vi "GSP_Manager_COLL.vi"() -> ()   [LabVIEW 2015]
uses:
  SystemUtil/ScriptArray.ctl
  SystemUtil/Script.ctl
  SystemUtil/Command.ctl
  SystemUtil/MotorStates.ctl
  SystemUtil/ThreadStates.ctl
  Log/LogItem.ctl
  GSP_COLL_Global.vi
  GUI/GSP_GUI_global.vi
panel:
  in  "Change Coll":bool
  out "Coll Actual":i32 caption="Actual"
  in  "Coll Target":i32 caption="Target" min=-4000 max=1000
  out "Coll Ext Temp":dbl(slide) scale=0.0..20.0
  out "Last Error":errorcluster
  in  "CommandQ":string
  # "Collimator Focus"
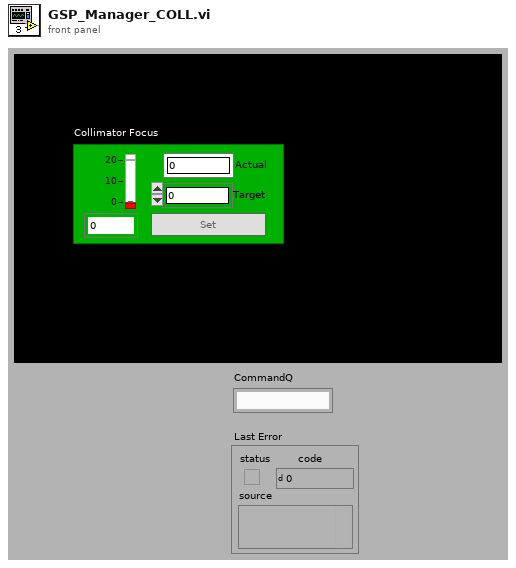
[diagram p1: front panel]
types:
  T1 = typedef "Command.ctl" = cluster{"Command":string, "Parameter":string}
  T2 = typedef "ScriptArray.ctl" = T3[]
  T3 = typedef "Script.ctl" = cluster{"Current Step":i32, "Commands":cluster{"Command":string, "Parameters":string}[]}
  T4 = cluster{"Move Mem Address":i32, "Home Mem Address":i32}
  T5 = enum16{"POL (0)", "CPL (1)", "HLT (2)", "STP (3)", "RST (4)", "RVN (5)", "RPB (6)", "CLP (8)", "SDL (9)", "RUN (10)", "WRI (11)", "RRG (12)", "SPR (13)", "LPR (14)", "VMI (15)", "SSP (17)", "SSE (18)", "RIS (20)", "RIO (21)", "IMW (25)", "END (128)", "MAV (134)", "MRV (135)", "JRE (137)", "WCL (138)", "WCW (139)", "DLY (140)", "WDL (141)", "GCL (142)", "GOP (143)", "ZTG (144)", "ZTP (145)", "TTP (146)", "CME (147)", "CTC (148)", "TQL (149)", "AHC (150)", "ERL (151)", "OLP (152)", "WRP (154)", "IDT (155)", "LRP (156)", "VMP (159)", "RAV (160)", "RRV (161)", "JMP (162)", "JOI (162)", "CIS (163)", "CKS (164)", "CLC (165)", "KMC (167)", "MCT (168)", "FLC (169)", "EEM (170)", "DDB (171)", "DEM (171)", "PAC (172)", "ADL (173)", "BRT (174)", "MAT (176)", "MRT (177)", "RAT (178)", "RRT (179)", "SSD (180)", "KMR (181)", "KED (182)", "KDD (183)", "DIR (184)", "PRO (185)", "SIF (186)", "EDL (187)", "CIO (188)", "MDS (189)", "MDC (190)", "MDT (191)", "SEE (192)", "ARI (193)", "WBS (194)", "SCF (195)", "RSM (196)", "RLM (197)", "RSN (198)", "RLN (199)", "PCL (201)", "PCI (201)", "PRT (202)", "PRI (202)", "WBE (204)", "SOB (205)", "COB (206)", "ACR (207)", "PLR (208)", "CAI (211)", "LVT (212)", "OVT (213)", "MTT (214)", "CLC (215)", "PIM (216)", "VIM (217)", "TIM (218)", "AHM (219)", "SSL (221)", "TRU (222)", "RSD (223)", "EMT (225)", "DMT (226)", "EMD (227)", "DMD (228)", "HSM (229)", "AHD (230)", "PCM (231)", "PCG (232)", "XRV (233)", "XAV (234)", "XRT (235)", "XAT (236)", "GOC (237)", "JNA (238)", "JOR (239)", "PMC (240)", "PMV (241)", "PMX (242)", "DLC (243)", "SLC (244)", "PCP (245)", "ATR (248)", "PMO (249)", "JAN (250)", "EDH (251)", "DIF (252)", "IMS (253)", "IMQ (254)"}
  T6 = typedef "MotorStates.ctl" = enum16{"Ready", "Moving", "Uninitialized", "Error"}
  T7 = typedef "ThreadStates.ctl" = enum16{"Waiting", "Scripting", "Uninitialized", "Error"}
  T8 = enum16{"Launch", "Log", "Open", "Close", "Shutdown"}
  T9 = typedef "LogItem.ctl" = cluster{"error in (no error)":errorcluster, "Source":string, "Comment ":string}
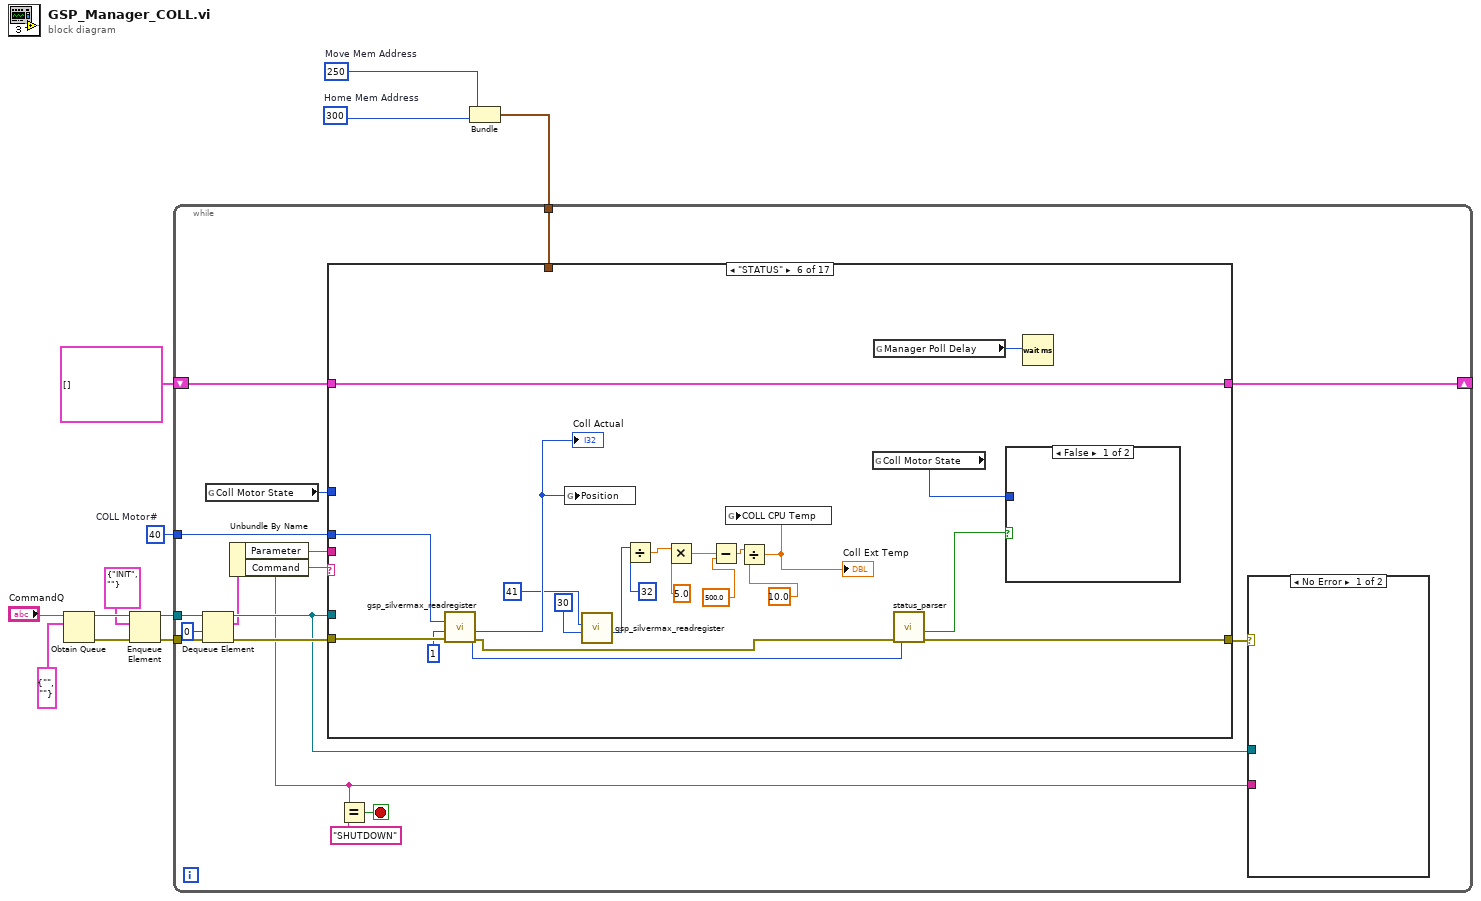
[diagram p0: block diagram]
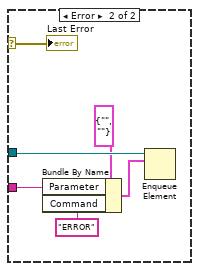
[diagram p2: hidden frame]
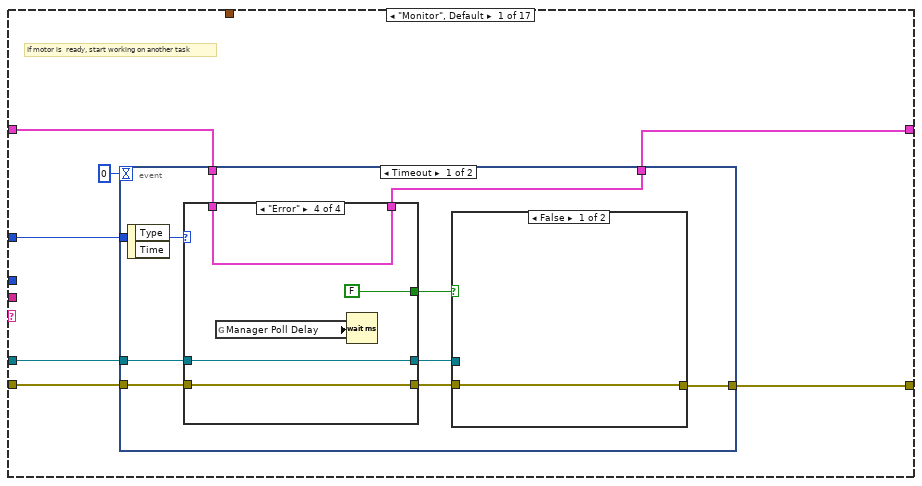
[diagram p3: hidden frame]
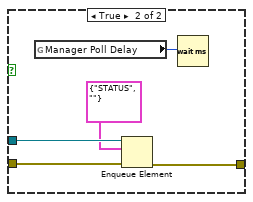
[diagram p4: hidden frame]
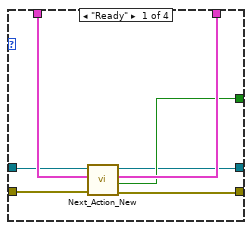
[diagram p5: hidden frame]
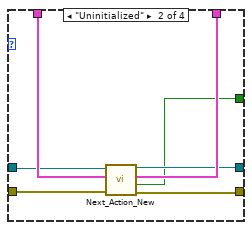
[diagram p6: hidden frame]
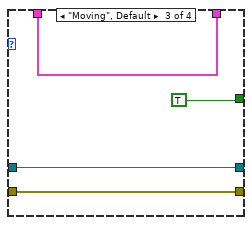
[diagram p7: hidden frame]
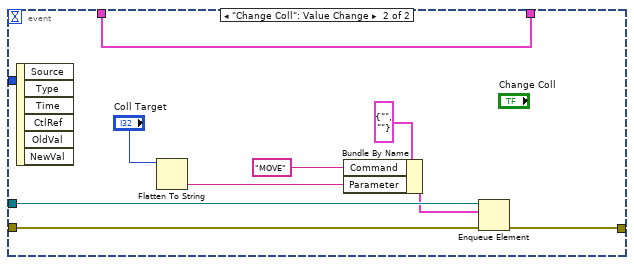
[diagram p8: hidden frame]
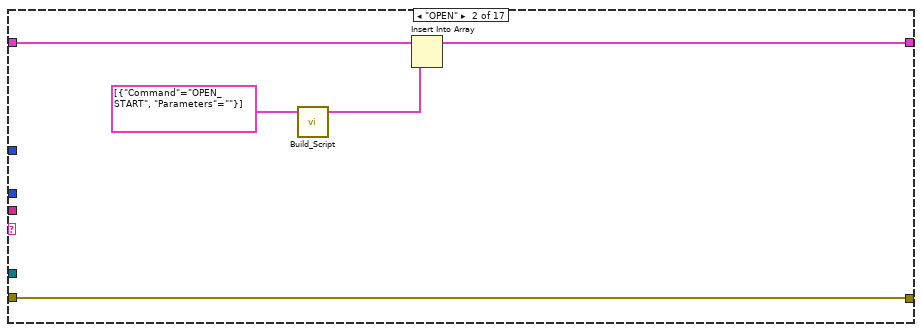
[diagram p9: hidden frame]
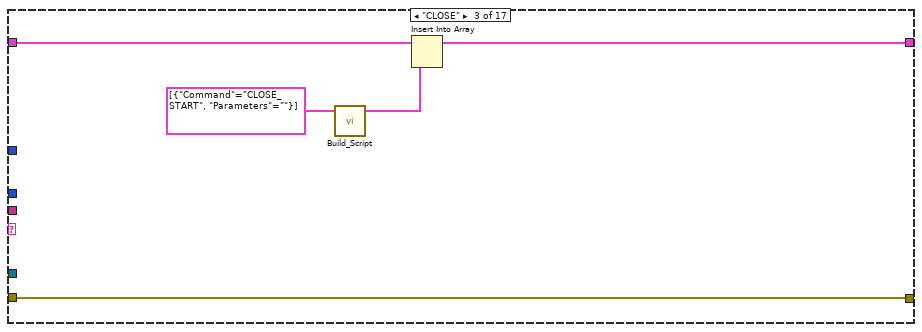
[diagram p10: hidden frame]
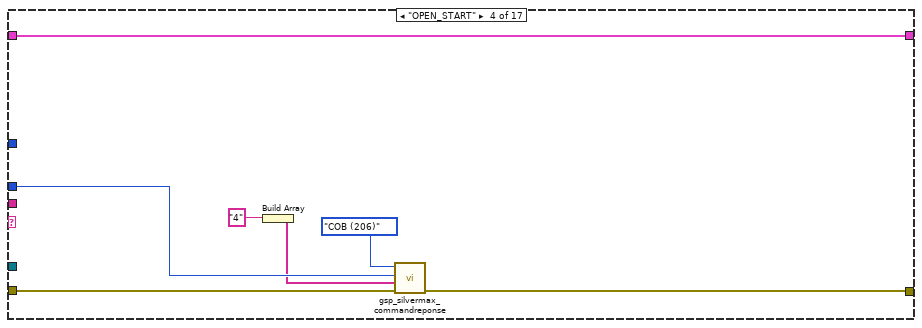
[diagram p11: hidden frame]
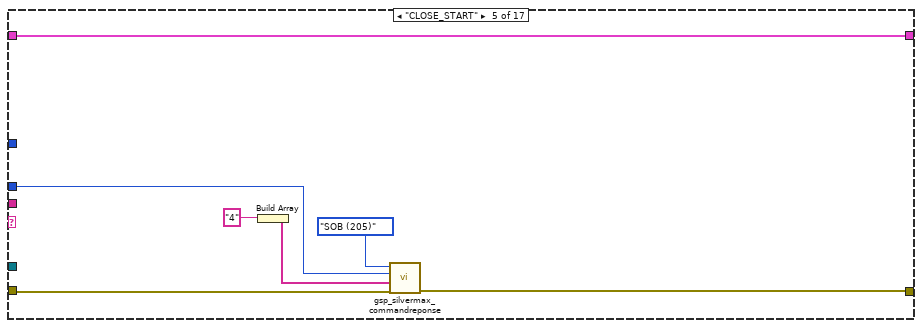
[diagram p12: hidden frame]
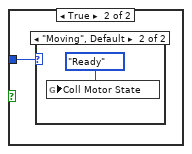
[diagram p13: hidden frame]
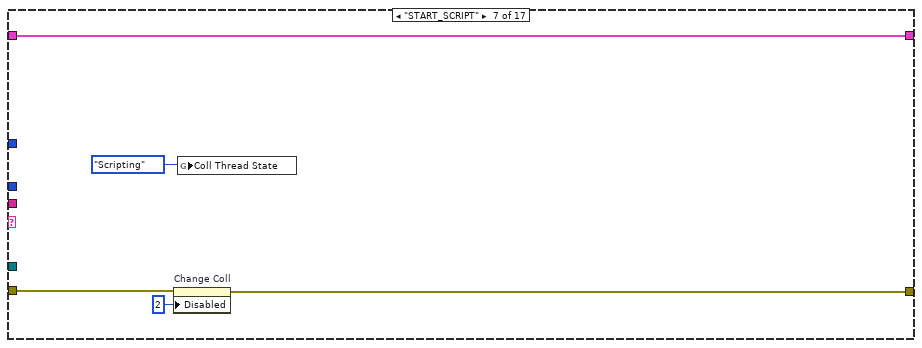
[diagram p15: hidden frame]
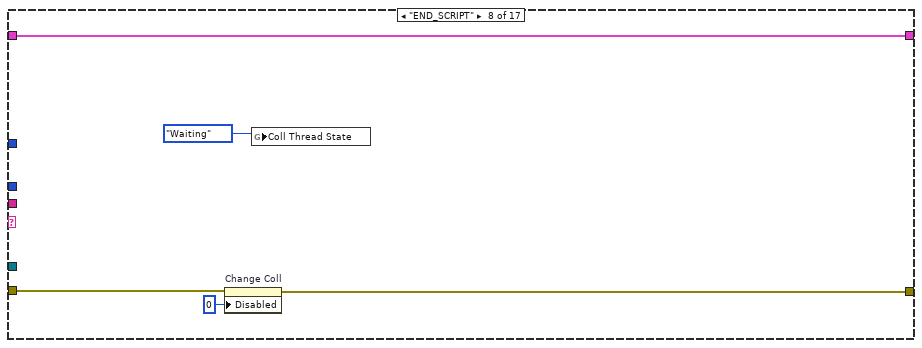
[diagram p16: hidden frame]
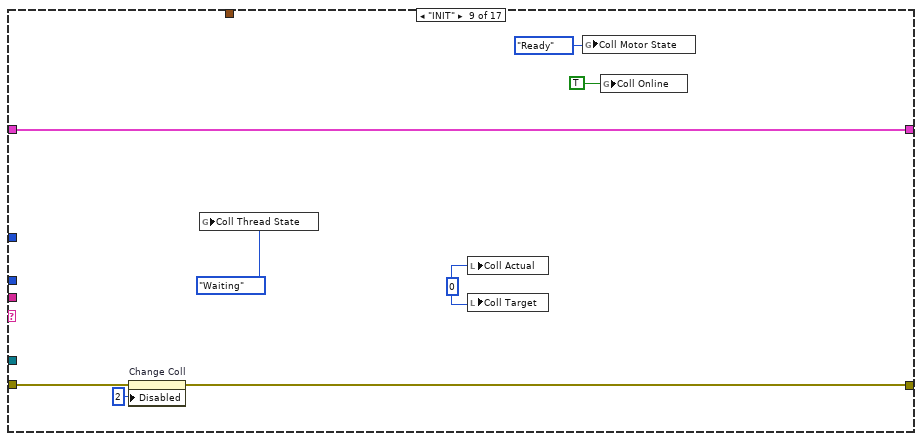
[diagram p17: hidden frame]
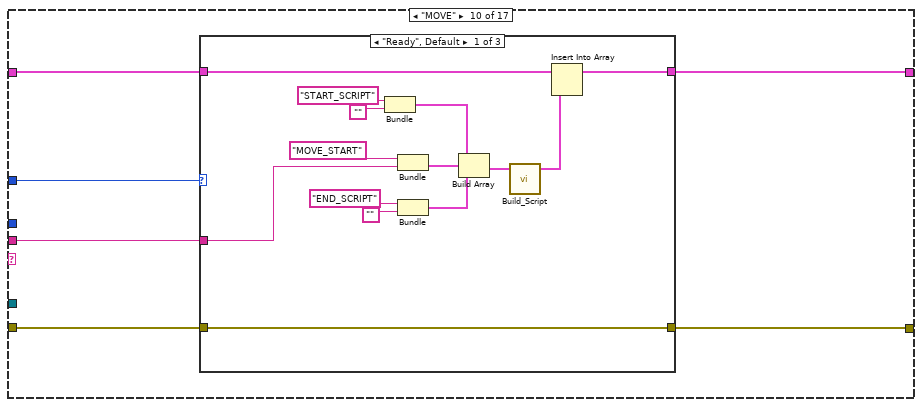
[diagram p18: hidden frame]
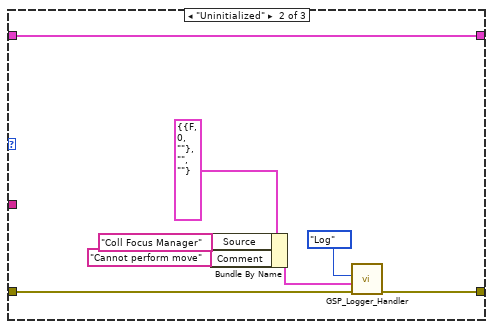
[diagram p19: hidden frame]
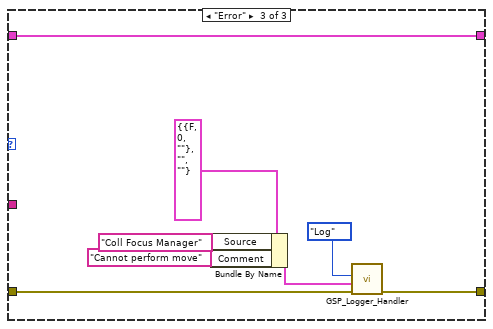
[diagram p20: hidden frame]
diagram:
  w2 = 300  # Home Mem Address
  w3 = 250  # Move Mem Address
  w4 = u8 40  # COLL Motor#
  n1 = Obtain Queue(name (unnamed)="CommandQ", element data type=T1 {"Command"="", "Parameter"=""} ("Command")) -> (queue out=w9:refnum<queue>, error out=w10:errorcluster)  [unwired: 3 in, 1 out]
  n2 = Enqueue Element(queue=w9, element=T1 {"Command"="INIT", "Parameter"=""}, error in (no error)=w10) -> (queue out=w12:refnum<queue>, error out=w11:errorcluster)  [unwired: 1 in, 1 out]
  n3 = Bundle("Move Mem Address"=w3, "Home Mem Address"=w2) -> (w1:T4)  [unwired: 1 in]
  n4 = while {
    tunnel: w12 -> [w28]
    tunnel: w11 -> [w27]
    tunnel: w4 -> [w22]
    shift-right: [w21] -> _
    shift-left: T2 [] ("Operations") -> [w20]
    tunnel: w1 -> [w13]
    stop <- w16 stop-if-true
    n5 = Dequeue Element(queue=w28, timeout in ms (-1)=0, error in (no error)=w27) -> (queue out=w24:refnum<queue>, element=w18:T1, error out=w26:errorcluster)  [unwired: 1 out]
    n6 = global read "GSP_COLL_Global.vi" "Coll Motor State"() -> (w14:T6)
    n7 = Unbundle By Name(w18) -> ("Parameter"=w17:string, "Command"=w15:string)
    n8 = case shown="\"STATUS\"" w15 {
      tunnel: w26 -> [w40 w91 w96 w104 w108 w134 w140 w145 w151 w157 w191 w214 w220 w223 w238 w242 _]
      tunnel: w24 -> [w41 _ _ _ _ _ _ _ _ _ _ w215 _ _ _ _ w251]
      tunnel: [w36 w91 w96 w102 w107 w131 w138 w143 w147 w156 w201 w212 w220 w229 w237 w241 _] -> w25
      tunnel: w22 -> [_ _ _ w100 w106 w133 _ _ _ _ w195 _ _ w232 _ _ _]
      tunnel: w20 -> [w39 w93 w98 w105 w112 w129 w141 w146 w153 w160 w198 w216 w222 w226 w239 w243 w246]
      tunnel: [w38 w92 w97 w105 w112 w129 w141 w146 w153 w159 w198 w216 w221 w226 w239 w243 w245] -> w21
      tunnel: w17 -> [_ _ _ _ _ _ _ _ _ w158 w196 _ _ _ _ _ _]
      tunnel: w14 -> [w37 _ _ _ _ _ _ _ _ w155 _ _ _ _ _ _ _]
      tunnel: w13 -> [_ _ _ _ _ _ _ _ _ _ w194 _ _ w225 _ _ _]
      frame "Monitor", Default {
        # "If motor is  ready, start working on another task"
        n9 = event shown="[0] Timeout" {
          selector: _ -> [_ _]
          dyn-events: _ -> [_ _]
          timeout: 0 -> [_ _]
          tunnel: w41 -> [w50 w83]
          tunnel: w40 -> [w49 w82]
          tunnel: w39 -> [w48 w88]
          tunnel: [w47 w88] -> w38
          tunnel: w37 -> [w46 _]
          tunnel: [w43 w81] -> w36
          event Timeout {
            n10 = event-data() -> ()  [unwired: 1 in, 2 out]
            n11 = case shown="\"Error\"" w46 {
              tunnel: w50 -> [w59 w66 w72 w76]
              tunnel: w49 -> [w63 w70 w73 w78]
              tunnel: [w61 w68 w73 w78] -> w45
              tunnel: w48 -> [w62 w69 w74 w79]
              tunnel: [w60 w67 w74 w79] -> w47
              tunnel: [w57 w65 w72 w76] -> w44
              tunnel: [w58 w64 TRUE FALSE] -> w42
              frame "Ready" {
                n12 = call "Next_Action_New.vi"("error in (no error)"=w63, "Operations"=w62, "queue in"=w59) -> ("error out"=w61:errorcluster, "No command?"=w58:bool, "Operations Out"=w60:T2, "queue out"=w57:refnum<queue>)  [unwired: 1 in]
              }
              frame "Uninitialized" {
                n13 = call "Next_Action_New.vi"("error in (no error)"=w70, "Operations"=w69, "queue in"=w66) -> ("error out"=w68:errorcluster, "No command?"=w64:bool, "Operations Out"=w67:T2, "queue out"=w65:refnum<queue>)  [unwired: 1 in]
              }
              frame "Moving", Default {
              }
              frame "Error" {
                n14 = global read "GSP_GUI_global.vi" "Manager Poll Delay"() -> (w77:u32)
                n15 = Wait (ms)(milliseconds to wait=w77) -> ()  [unwired: 1 out]
              }
            }
            n16 = case shown="False" w42 {
              tunnel: w45 -> [w51 w56]
              tunnel: w44 -> [_ w55]
              tunnel: [w51 w54] -> w43
              frame False {
              }
              frame True {
                n17 = global read "GSP_GUI_global.vi" "Manager Poll Delay"() -> (w53:u32)
                n18 = Enqueue Element(queue=w55, element=T1 {"Command"="STATUS", "Parameter"=""}, error in (no error)=w56) -> (error out=w54:errorcluster)  [unwired: 1 in, 2 out]
                n19 = Wait (ms)(milliseconds to wait=w53) -> ()  [unwired: 1 out]
              }
            }
          }
          event "Change Coll": Value Change {
            n20 = event-data() -> ()  [unwired: 1 in, 6 out]
            n21 = Flatten To String(anything="Coll Target") -> (data string=w85:string)  [unwired: 3 in, 2 out]
            n22 = Bundle By Name(cluster=T1 {"Command"="", "Parameter"=""} ("element"), "Command"="MOVE" ("element"), "Parameter"=w85) -> (w80:T1)
            n23 = Enqueue Element(queue=w83, element=w80, error in (no error)=w82) -> (error out=w81:errorcluster)  [unwired: 1 in, 2 out]
          }
        }
      }
      frame "OPEN" {
        n24 = call "Build_Script.vi"("Commands"=cluster{"Command":string, "Parameters":string}[] [{"Command"="OPEN_START", "Parameters"=""}]) -> ("script out"=w90:T3)  [unwired: 4 in]
        n25 = Insert Into Array(array=w93, new element=w90) -> (w92:T2)  [unwired: 1 in]
      }
      frame "CLOSE" {
        n26 = call "Build_Script.vi"("Commands"=cluster{"Command":string, "Parameters":string}[] [{"Command"="CLOSE_START", "Parameters"=""}]) -> ("script out"=w95:T3)  [unwired: 4 in]
        n27 = Insert Into Array(array=w98, new element=w95) -> (w97:T2)  [unwired: 1 in]
      }
      frame "OPEN_START" {
        n28 = Build Array("4") -> (w99:string[])
        n29 = call "gsp_silvermax_commandreponse.vi"("error in (no error)"=w104, "Parameters (none)"=w99, "Motor #"=w100, "Command"=T5."COB (206)") -> ("error out"=w102:errorcluster)  [unwired: 3 out]
      }
      frame "CLOSE_START" {
        n30 = Build Array("4") -> (w109:string[])
        n31 = call "gsp_silvermax_commandreponse.vi"("error in (no error)"=w108, "Parameters (none)"=w109, "Motor #"=w106, "Command"=T5."SOB (205)") -> ("error out"=w107:errorcluster)  [unwired: 3 out]
      }
      frame "STATUS" {
        n32 = call "gsp_silvermax_readregister.vi"("error in (no error)"=w134, "Register# (0)"=u8 1, "Motor #"=w133) -> ("error out"=w113:errorcluster, "Register Value"=w121:i32, "Motor # dup"=w114:u8)  [unwired: 2 in, 2 out]
        "Coll Actual" <- w121
        n33 = global write "GSP_COLL_Global.vi" "Position"(w121) -> ()
        n34 = call "gsp_silvermax_readregister.vi"("Register# (0)"=u8 30, "Motor #"=41) -> ("Register Value"=w123:i32)  [unwired: 3 in, 4 out]
        n35 = Divide(x=w123, y=32) -> (x/y=w125:dbl)
        n36 = Multiply(x=w125, y=5.0) -> (x*y=w120:dbl)
        n37 = Subtract(x=w120, y=500.0) -> (x-y=w119:dbl)
        n38 = Divide(x=w119, y=10.0) -> (x/y=w117:dbl)
        "Coll Ext Temp" <- w117
        n39 = global write "GSP_COLL_Global.vi" "COLL CPU Temp"(w117) -> ()
        n40 = global read "GSP_COLL_Global.vi" "Coll Motor State"() -> (w122:T6)
        n41 = global read "GSP_GUI_global.vi" "Manager Poll Delay"() -> (w128:u32)
        n42 = call "status_parser.vi"("error in (no error)"=w113, "Motor #"=w114) -> ("error out"=w131:errorcluster, "Program Complete?"=w130:bool)  [unwired: 3 in, 1 out]
        n43 = case shown="False" w130 {
          tunnel: w122 -> [_ w135]
          frame False {
          }
          frame True {
            n44 = case shown="\"Moving\", Default" w135 {
              frame "Uninitialized" {
              }
              frame "Moving", Default {
                n45 = global write "GSP_COLL_Global.vi" "Coll Motor State"(MotorStates."Ready" ("Mode")) -> ()
              }
            }
          }
        }
        n46 = Wait (ms)(milliseconds to wait=w128) -> ()  [unwired: 1 out]
      }
      frame "START_SCRIPT" {
        n47 = property on="Change Coll" class="Bool"(error in=w140, "Disabled"=u8 2) -> (error out=w138:errorcluster)  [unwired: 1 in, 1 out]
        n48 = global write "GSP_COLL_Global.vi" "Coll Thread State"(ThreadStates."Scripting" ("Thread state")) -> ()
      }
      frame "END_SCRIPT" {
        n49 = property on="Change Coll" class="Bool"(error in=w145, "Disabled"=u8 0) -> (error out=w143:errorcluster)  [unwired: 1 in, 1 out]
        n50 = global write "GSP_COLL_Global.vi" "Coll Thread State"(ThreadStates."Waiting" ("Thread state")) -> ()
      }
      frame "INIT" {
        w150 = 0 ("Value")
        n51 = property on="Change Coll" class="Bool"(error in=w151, "Disabled"=u8 2) -> (error out=w147:errorcluster)  [unwired: 1 in, 1 out]
        n52 = global write "GSP_COLL_Global.vi" "Coll Thread State"(ThreadStates."Waiting" ("Thread state")) -> ()
        n53 = local write "Coll Actual"(w150) -> ()
        n54 = local write "Coll Target"(w150) -> ()
        n55 = global write "GSP_COLL_Global.vi" "Coll Motor State"(MotorStates."Ready" ("Mode")) -> ()
        n56 = global write "GSP_COLL_Global.vi" "Coll Online"(TRUE ("CS Online")) -> ()
      }
      frame "MOVE" {
        n57 = case shown="\"Ready\", Default" w155 {
          tunnel: w160 -> [w174 w176 w184]
          tunnel: [w173 w176 w184] -> w159
          tunnel: w158 -> [w167 _ _]
          tunnel: w157 -> [w172 w182 w190]
          tunnel: [w172 w181 w189] -> w156
          frame "Ready", Default {
            n58 = Bundle("START_SCRIPT", "") -> (w161:cluster{string, string})  [unwired: 1 in]
            n59 = Bundle("MOVE_START", "Parameter"=w167) -> (w166:cluster{string, "Parameter":string})  [unwired: 1 in]
            n60 = Bundle("END_SCRIPT", "") -> (w165:cluster{string, string})  [unwired: 1 in]
            n61 = Build Array(w161, w166, w165) -> (w164:cluster{string, "Parameter":string}[])
            n62 = call "Build_Script.vi"("Commands"=w164) -> ("script out"=w171:T3)  [unwired: 4 in]
            n63 = Insert Into Array(array=w174, new element=w171) -> (w173:T2)  [unwired: 1 in]
          }
          frame "Uninitialized" {
            n64 = Bundle By Name(cluster=T9 {"error in (no error)"={"status"=FALSE, "code"=0, "source"=""}, "Source"="", "Comment "=""} ("Log"), "Source"="Coll Focus Manager", "Comment"="Cannot perform move") -> (w180:T9)
            n65 = call "GSP_Logger_Handler.vi"("error in (no error)"=w182, "Log"=w180, "Actions"=T8."Log") -> ("error out"=w181:errorcluster)  [unwired: 4 in]
          }
          frame "Error" {
            n66 = Bundle By Name(cluster=T9 {"error in (no error)"={"status"=FALSE, "code"=0, "source"=""}, "Source"="", "Comment "=""} ("Log"), "Source"="Coll Focus Manager", "Comment"="Cannot perform move") -> (w188:T9)
            n67 = call "GSP_Logger_Handler.vi"("error in (no error)"=w190, "Log"=w188, "Actions"=T8."Log") -> ("error out"=w189:errorcluster)  [unwired: 4 in]
          }
        }
      }
      frame "MOVE_START" {
        n68 = Unflatten From String(type=0, binary string=w196) -> (value=w192:i32)  [unwired: 3 in, 2 out]
        n69 = Unbundle By Name(w194) -> ("Move Mem Address"=w193:i32)
        n70 = local write "Coll Target"(w192) -> ()
        n71 = global write "GSP_COLL_Global.vi" "Target"(w192) -> ()
        n72 = Number To Decimal String(number=w193) -> (decimal integer string=w200:string)  [unwired: 1 in]
        n73 = call "gsp_silvermax_writeregister.vi"("error in (no error)"=w191, "Register Value"=w192, "Motor #"=w195, "Register# (0)"=u8 25) -> ("error out"=w205:errorcluster, "Motor # dup"=w203:u8)  [unwired: 2 in]
        n74 = Build Array(w200) -> (w199:string[])
        n75 = call "gsp_silvermax_commandreponse.vi"("error in (no error)"=w205, "Parameters (none)"=w199, "Motor #"=w203, "Command"=T5."LRP (156)") -> ("error out"=w202:errorcluster)  [unwired: 3 out]
        n76 = case shown="No Error" w202 {
          selector: w202 -> [w208 w209]
          tunnel: [w208 w209] -> w201
          frame No Error {
            n77 = global write "GSP_COLL_Global.vi" "Coll Motor State"(MotorStates."Moving" ("Mode")) -> ()
          }
          frame Error {
          }
        }
      }
      frame "SHUTDOWN" {
        n78 = Release Queue(queue=w215, error in (no error)=w214) -> (error out=w211:errorcluster)  [unwired: 1 in, 2 out]
        n79 = global write "GSP_COLL_Global.vi" "Coll Thread State"(ThreadStates."Uninitialized" ("Thread state")) -> ()
        n80 = property on="Change Coll" class="Bool"(error in=w211, "Disabled"=u8 2) -> (error out=w212:errorcluster)  [unwired: 1 in, 1 out]
        n81 = stacked-sequence {
          tunnel: w212 -> [_]
          frame #0 {
            n82 = global write "GSP_COLL_Global.vi" "Coll Online"(FALSE ("CS Online")) -> ()
          }
        }
      }
      frame "HOME" {
        n83 = call "Build_Script.vi"("Commands"=cluster{"Command":string, "Parameters":string}[] [{"Command"="START_SCRIPT", "Parameters"=""}, {"Command"="HOME_START", "Parameters"=""}, {"Command"="END_SCRIPT", "Parameters"=""}]) -> ("script out"=w218:T3)  [unwired: 4 in]
        n84 = Insert Into Array(array=w222, new element=w218) -> (w221:T2)  [unwired: 1 in]
      }
      frame "HOME_START" {
        n85 = Unbundle By Name(w225) -> ("Home Mem Address"=w224:i32)
        n86 = Number To Decimal String(number=w224) -> (decimal integer string=w228:string)  [unwired: 1 in]
        n87 = Build Array(w228) -> (w227:string[])
        n88 = call "gsp_silvermax_commandreponse.vi"("error in (no error)"=w223, "Parameters (none)"=w227, "Motor #"=w232, "Command"=T5."LRP (156)") -> ("error out"=w230:errorcluster)  [unwired: 3 out]
        n89 = case shown="No Error" w230 {
          selector: w230 -> [w234 w235]
          tunnel: [w234 w235] -> w229
          frame No Error {
            n90 = global write "GSP_COLL_Global.vi" "Coll Motor State"(MotorStates."Moving" ("Mode")) -> ()
          }
          frame Error {
          }
        }
      }
      frame "DISABLE" {
        n91 = property on="Change Coll" class="Bool"(error in=w238, "DisabledEnum"=2) -> (error out=w237:errorcluster)  [unwired: 1 in, 1 out]
      }
      frame "ENABLE" {
        n92 = property on="Change Coll" class="Bool"(error in=w242, "DisabledEnum"=0) -> (error out=w241:errorcluster)  [unwired: 1 in, 1 out]
      }
      frame "ERROR" {
        n93 = local read "Last Error"() -> (w247:errorcluster)
        n94 = Unbundle By Name(w247) -> ("code"=w253:i32)
        n95 = Bundle By Name(cluster=T9 {"error in (no error)"={"status"=FALSE, "code"=0, "source"=""}, "Source"="", "Comment "=""} ("Log"), "error in (no error)"=w247, "Source"="Coll Manager") -> (w248:T9)
        n96 = call "GSP_Logger_Handler.vi"("Log"=w248, "Actions"=T8."Log") -> ()  [unwired: 5 in, 1 out]
        n97 = case shown="0, Default" w253 {
          tunnel: w247 -> [_ _ _ _]
          tunnel: [errorcluster {"status"=FALSE, "code"=0, "source"=""} ("Last Error") errorcluster {"status"=FALSE, "code"=0, "source"=""} ("Last Error") errorcluster {"status"=FALSE, "code"=0, "source"=""} ("Last Error") errorcluster {"status"=FALSE, "code"=0, "source"=""} ("Last Error")] -> w252
          tunnel: w246 -> [_ w262 w264 w266]
          tunnel: [T2 [] ("Operations") w262 w264 w266] -> w245
          frame 0, Default {
            n98 = global write "GSP_COLL_Global.vi" "Coll Motor State"(MotorStates."Error" ("Mode")) -> ()
            n99 = global write "GSP_COLL_Global.vi" "Coll Thread State"(ThreadStates."Error" ("Thread state")) -> ()
            n100 = property on="Change Coll" class="Bool"("Disabled"=u8 2) -> ()  [unwired: 2 in, 2 out]
          }
          frame 5003 {
          }
          frame 5006 {
          }
          frame 5013 {
          }
        }
        n101 = case shown="No Error" w252 {
          tunnel: w251 -> [_ w255]
          frame No Error {
          }
          frame Error {
            n102 = Enqueue Element At Opposite End(queue=w255, element=T1 {"Command"="SHUTDOWN", "Parameter"=""}) -> ()  [unwired: 2 in, 3 out]
          }
        }
      }
    }
    n103 = Equal?(x=w15, y="SHUTDOWN") -> (x = y?=w16:bool)
    n104 = case shown="No Error" w25 {
      selector: w25 -> [_ w33]
      tunnel: w24 -> [_ w34]
      tunnel: w15 -> [_ w31]
      frame No Error {
      }
      frame Error {
        n105 = Bundle By Name(cluster=T1 {"Command"="", "Parameter"=""} ("element"), "Parameter"=w31, "Command"="ERROR" ("element")) -> (w29:T1)
        n106 = Enqueue Element(queue=w34, element=w29) -> ()  [unwired: 2 in, 3 out]
        "Last Error" <- w33
      }
    }
  }
